vi "EcoSense.vi"() -> ()   [LabVIEW 2022 SP3]
uses:
  <vilib>/DAQmx/read.llb/DAQmx Read (Analog 1D DBL NChan 1Samp).vi
  <vilib>/DAQmx/write.llb/DAQmx Write (Digital Bool 1Line 1Point).vi
  <vilib>/DAQmx/create/channels.llb/DAQmx Create Channel (AI-Voltage-Basic).vi
  <vilib>/DAQmx/create/channels.llb/DAQmx Create Channel (DO-Digital Output).vi
  <vilib>/DAQmx/miscellaneous.llb/DAQmx Fill In Error Info.vi
panel:
  in  "Connect":bool
  in  "Write":bool
  in  "Read":bool
  in  "Exit":bool
  out "Return":string
  in  "byte count":u32
  in  "Command":string
  in  "VISA resource name":refnum<visa-resource-name>
  in  "lines 4 fire detection call":tag
  out "elapsed time":dbl
  out "PPM Meter":dbl(knob) scale=0.0..3000.0
  out "LP gas":bool
  out "CO2 gas":bool
  out "Low Temperature":bool
  out "Normal Temperature":bool
  out "HIgh Temperature":bool
  out "time":string
  out "date":string
  out "Exhaust Fan":bool
  out "Thermometer":dbl(slide) scale=0.0..100.0
  out "Temperature7 (C)":dbl
  in  "lines 3 Gas leakage call":tag
  in  "Manual Exhaust fan Switch":bool
  in  "Manual window close\n switch":bool
  out "rain":bool
  in  "lines 2 Rain sensor":tag
  out "Sensor in the bedroom 2":string
  out "Sensor in the master bedroom":string
  out "Sensor in the dining room":string
  out "Sensor in the living room":string
  out "Sensor in the kitchen":string
  in  "Manual Pump motor switch":bool
  out "Gas sensor6-(ppm)":dbl
  out "Fire":bool
  out "Gas Indicator":string
  out "Rain Sensor":dbl
  in  "lines 1 for Exhaust Fan":tag
  in  "lines 0 for Fire sensor":tag
  out "IRsensor5-Blue":dbl
  out "IR sensor1-Purple":dbl
  out "Irsensor4-Yellow":dbl
  out "IRsensor2-Green":dbl
  out "IRsensor0 - Orange":dbl
  in  "stop":bool
  in  "physical channels":tag
  # "Automated Home Wellness System"
  # "Fire Sensor"
  # "Gas Sensor"
  # "DC Power Supply"
  # "Gas Sensor6 - ppm"
  # "Thermometer"
  # "Exhuast Fan"
  # "Rain sensor indicator 3"
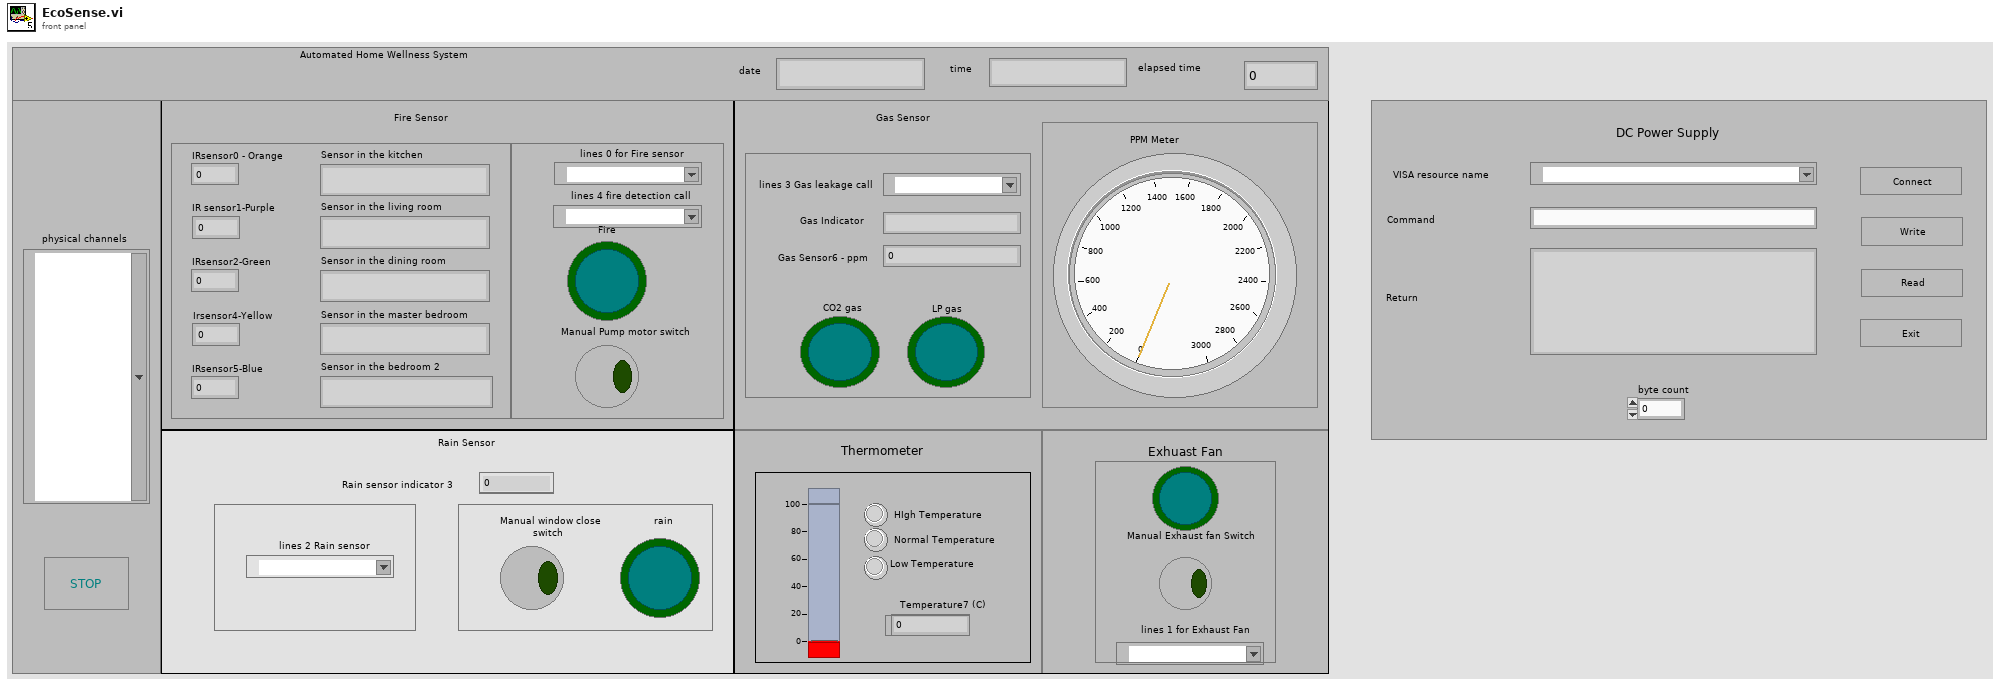
[diagram p1: front panel]
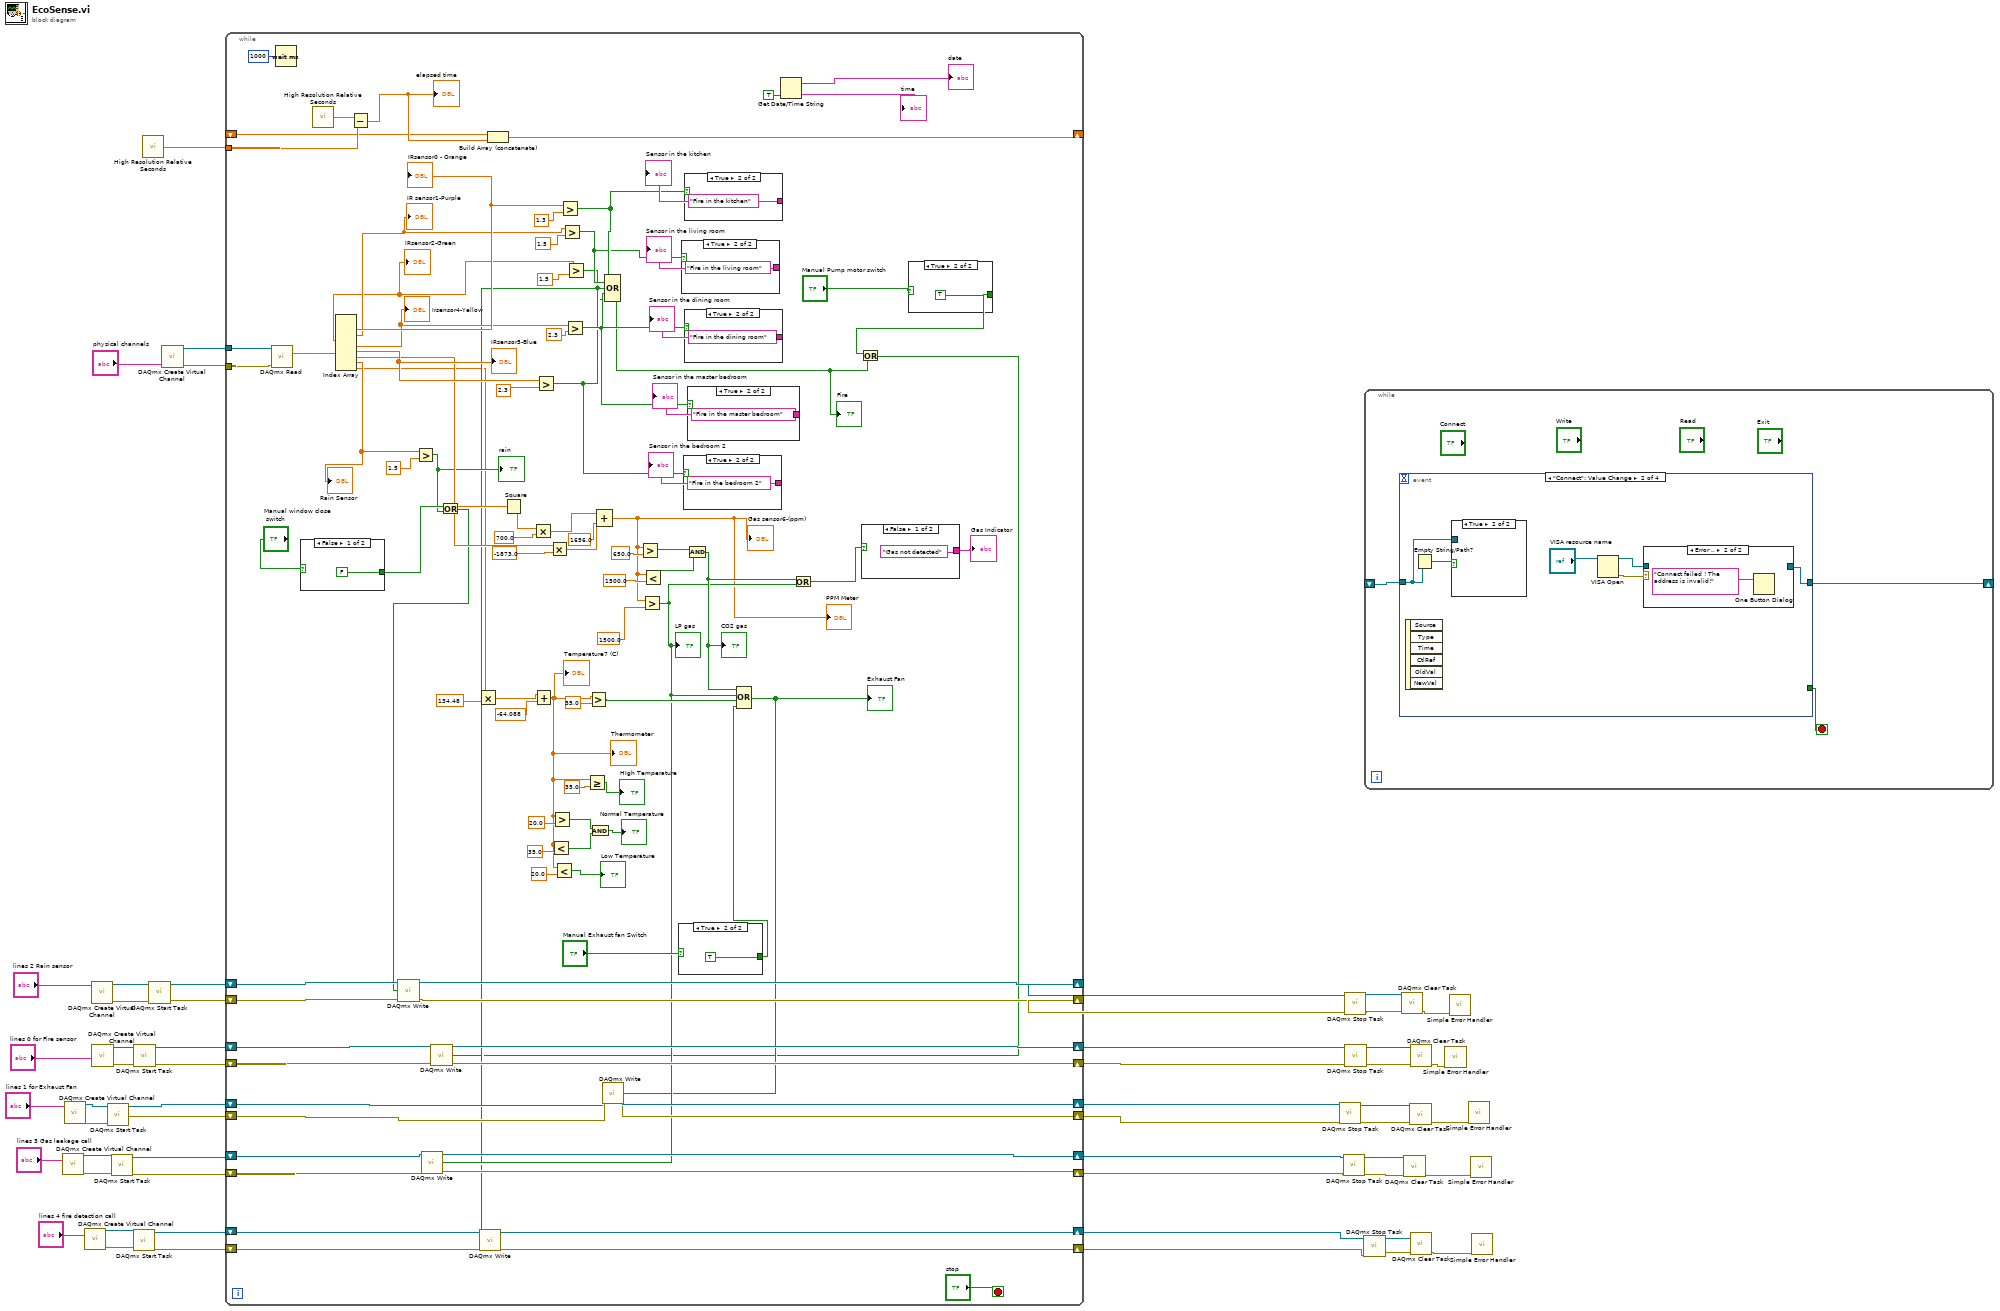
[diagram p0: block diagram]
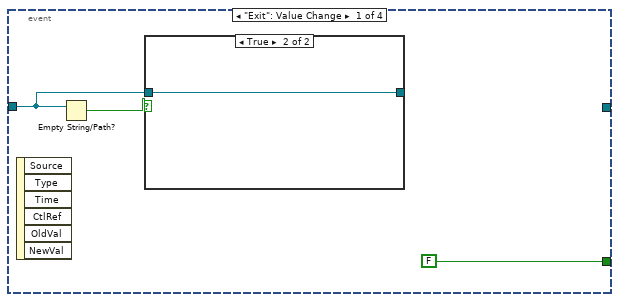
[diagram p2: hidden frame]
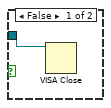
[diagram p5: hidden frame]
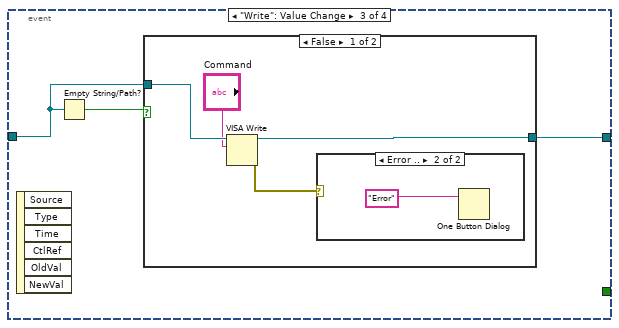
[diagram p6: hidden frame]
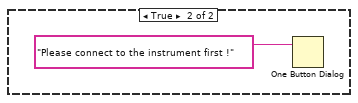
[diagram p8: hidden frame]
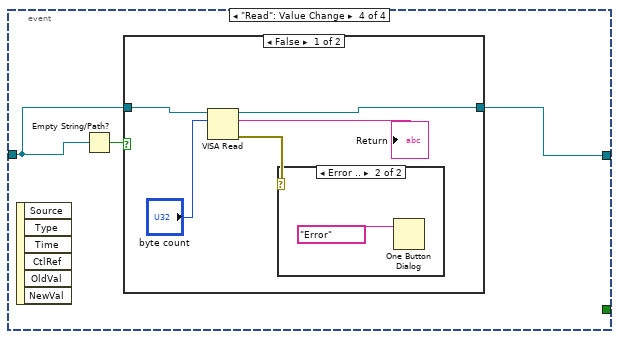
[diagram p9: hidden frame]
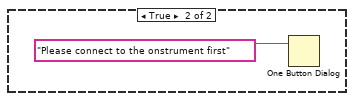
[diagram p11: hidden frame]
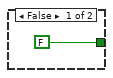
[diagram p12: hidden frame]
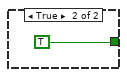
[diagram p13: hidden frame]
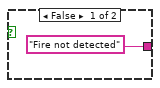
[diagram p14: hidden frame]
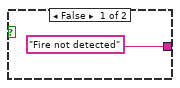
[diagram p15: hidden frame]
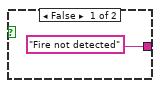
[diagram p16: hidden frame]
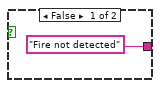
[diagram p17: hidden frame]
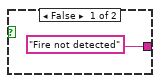
[diagram p18: hidden frame]
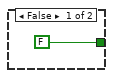
[diagram p19: hidden frame]
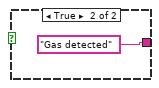
[diagram p20: hidden frame]
diagram:
  n1 = call-poly <vilib>:"DAQmx Create Virtual Channel.vi"("lines"="lines 3 Gas leakage call") -> ("task out"=w19:refnum<k21>, "error out"=w18:errorcluster)  [unwired: 13 in]
  n2 = call-poly <vilib>:"DAQmx Create Virtual Channel.vi"("lines"="lines 1 for Exhaust Fan") -> ("task out"=w43:refnum<k21>, "error out"=w27:errorcluster)  [unwired: 13 in]
  n3 = call-poly <vilib>:"DAQmx Create Virtual Channel.vi"("lines"="lines 4 fire detection call") -> ("task out"=w9:refnum<k21>, "error out"=w8:errorcluster)  [unwired: 13 in]
  n4 = call-poly <vilib>:"DAQmx Create Virtual Channel.vi"("lines"="lines 2 Rain sensor") -> ("task out"=w32:refnum<k21>, "error out"=w29:errorcluster)  [unwired: 13 in]
  n5 = call-poly <vilib>:"DAQmx Create Virtual Channel.vi"("lines"="lines 0 for Fire sensor") -> ("task out"=w50:refnum<k21>, "error out"=w28:errorcluster)  [unwired: 13 in]
  n6 = call <vilib>:"DAQmx Start Task.vi"("task/channels in"=w43, "error in"=w27) -> ("task out"=w41:refnum<k21>, "error out"=w42:errorcluster)  [unwired: 12 in]
  n7 = call <vilib>:"DAQmx Start Task.vi"("task/channels in"=w19, "error in"=w18) -> ("task out"=w17:refnum<k21>, "error out"=w16:errorcluster)  [unwired: 12 in]
  n8 = call <vilib>:"DAQmx Start Task.vi"("task/channels in"=w9, "error in"=w8) -> ("task out"=w7:refnum<k21>, "error out"=w6:errorcluster)  [unwired: 12 in]
  n9 = call <vilib>:"DAQmx Start Task.vi"("task/channels in"=w50, "error in"=w28) -> ("task out"=w46:refnum<k21>, "error out"=w35:errorcluster)  [unwired: 12 in]
  n10 = call <vilib>:"High Resolution Relative Seconds.vi"() -> ("relative seconds"=w34:dbl)
  n11 = call <vilib>:"DAQmx Start Task.vi"("task/channels in"=w32, "error in"=w29) -> ("task out"=w31:refnum<k21>, "error out"=w30:errorcluster)  [unwired: 12 in]
  n12 = call-poly <vilib>:"DAQmx Create Virtual Channel.vi"("physical channels"="physical channels") -> ("task out"=w52:refnum<k21>, "error out"=w53:errorcluster)  [unwired: 13 in]
  n13 = while {
    tunnel: w53 -> [w147]
    tunnel: w52 -> [w153]
    tunnel: w34 -> [w151]
    shift-right: [w146] -> _
    shift-left: _ -> [w148]
    shift-right: [w141] -> w47
    shift-left: w46 -> [w142]
    shift-right: [w139] -> w45
    shift-left: w35 -> [w140]
    shift-right: [w131] -> w40
    shift-left: w41 -> [w128]
    shift-right: [w129] -> w39
    shift-left: w42 -> [w130]
    shift-right: [w99] -> w25
    shift-left: w31 -> [w100]
    shift-right: [w97] -> w26
    shift-left: w30 -> [w98]
    shift-right: [w81] -> w15
    shift-left: w17 -> [w82]
    shift-right: [w80] -> w14
    shift-left: w16 -> [w83]
    shift-right: [w61] -> w5
    shift-left: w7 -> [w63]
    shift-right: [w60] -> w1
    shift-left: w6 -> [w62]
    stop <- "stop" stop-if-true
    n14 = call-poly <vilib>:"DAQmx Read.vi"("task/channels in"=w153, "error in"=w147) -> ("data"=w145:dbl[])  [unwired: 11 in, 2 out]
    n15 = Wait (ms)(milliseconds to wait=u32 1000) -> ()  [unwired: 1 out]
    n16 = case shown="False" "Manual window close\n switch" {
      tunnel: [FALSE TRUE] -> w95
      frame False {
      }
      frame True {
      }
    }
    n17 = call <vilib>:"High Resolution Relative Seconds.vi"() -> ("relative seconds"=w150:dbl)
    n18 = Index Array(array=w145) -> (element #1=w144:dbl, element #2=w137:dbl, element #3=w57:dbl, element #4=w134:dbl, element #5=w132:dbl, element #6=w117:dbl, element #7=w96:dbl, element #8=w56:dbl)  [unwired: 8 in]
    "IRsensor0 - Orange" <- w144
    "IR sensor1-Purple" <- w137
    "IRsensor5-Blue" <- w132
    "IRsensor2-Green" <- w57
    "Irsensor4-Yellow" <- w134
    "Rain Sensor" <- w96
    n19 = Subtract(x=w150, y=w151) -> (x-y=w149:dbl)
    "elapsed time" <- w149
    n20 = Greater?(x=w96, y=1.5) -> (0:w66:bool)
    "rain" <- w66
    n21 = Or(x=w95, y=w66) -> (x .or. y?=w93:bool)
    n22 = call-poly <vilib>:"DAQmx Write.vi"("task/channels in"=w100, "data"=w93, "error in"=w98) -> ("task out"=w99:refnum<k21>, "error out"=w97:errorcluster)  [unwired: 10 in, 1 out]
    n23 = Multiply(x=w56, y=134.48) -> (x*y=w91:dbl)
    n24 = Build Array (concatenate)(w148, w149) -> (w146:dbl[])
    n25 = Square(x=w117) -> (x^2=w122:dbl)
    n26 = Multiply(x=w122, y=700.0) -> (x*y=w115:dbl)
    n27 = Add(x=w91, y=-64.088) -> (x+y=w55:dbl)
    "Temperature7 (C)" <- w55
    "Thermometer" <- w55
    n28 = Greater?(x=w132, y=2.3) -> (0:w101:bool)
    n29 = Multiply(x=w117, y=-1873.0) -> (x*y=w114:dbl)
    n30 = Less?(x=w55, y=35.0) -> (x < y?=w70:bool)
    n31 = Greater?(x=w55, y=20.0) -> (0:w71:bool)
    n32 = Less?(x=w55, y=20.0) -> (x < y?=→"Low Temperature":bool)
    n33 = Greater?(x=w144, y=1.3) -> (0:w108:bool)
    n34 = Greater?(x=w137, y=1.5) -> (0:w107:bool)
    n35 = Greater?(x=w134, y=2.3) -> (0:w103:bool)
    n36 = Greater?(x=w57, y=1.5) -> (0:w105:bool)
    n37 = Greater Or Equal?(x=w55, y=35.0) -> (x >= y?=→"HIgh Temperature":bool)
    n38 = Greater?(x=w55, y=35.0) -> (0:w88:bool)
    n39 = And(x=w71, y=w70) -> (x .and. y?=→"Normal Temperature":bool)
    n40 = Compound Arithmetic op=ADD(w115, w114, 1656.0 ("value")) -> (w65:dbl)
    "Gas sensor6-(ppm)" <- w65
    "PPM Meter" <- w65
    n41 = Compound Arithmetic op=OR(w108, w107, w105, w103, w101) -> (w59:bool)
    "Fire" <- w59
    n42 = call-poly <vilib>:"DAQmx Write.vi"("task/channels in"=w63, "data"=w59, "error in"=w62) -> ("task out"=w61:refnum<k21>, "error out"=w60:errorcluster)  [unwired: 10 in, 1 out]
    n43 = Greater?(x=w65, y=650.0) -> (0:w127:bool)
    n44 = Greater?(x=w65, y=1500.0) -> (0:w79:bool)
    "LP gas" <- w79
    n45 = call-poly <vilib>:"DAQmx Write.vi"("task/channels in"=w82, "data"=w79, "error in"=w83) -> ("task out"=w81:refnum<k21>, "error out"=w80:errorcluster)  [unwired: 10 in, 1 out]
    n46 = Less?(x=w65, y=1500.0) -> (x < y?=w126:bool)
    n47 = case shown="True" "Manual Exhaust fan Switch" {
      tunnel: [FALSE TRUE] -> w86
      frame False {
      }
      frame True {
      }
    }
    n48 = case shown="True" w107 {
      tunnel: ["Fire not detected" "Fire in the living room"] -> w109
      frame False {
      }
      frame True {
      }
    }
    "Sensor in the living room" <- w109
    n49 = case shown="True" w101 {
      tunnel: ["Fire not detected" "Fire in the bedroom 2"] -> w102
      frame False {
      }
      frame True {
      }
    }
    "Sensor in the bedroom 2" <- w102
    n50 = case shown="True" w105 {
      tunnel: ["Fire not detected" "Fire in the dining room"] -> w106
      frame False {
      }
      frame True {
      }
    }
    "Sensor in the dining room" <- w106
    n51 = case shown="True" w108 {
      tunnel: ["Fire not detected" "Fire in the kitchen"] -> w110
      frame False {
      }
      frame True {
      }
    }
    "Sensor in the kitchen" <- w110
    n52 = And(x=w127, y=w126) -> (x .and. y?=w85:bool)
    "CO2 gas" <- w85
    n53 = case shown="True" w103 {
      tunnel: ["Fire not detected" "Fire in the master bedroom"] -> w104
      frame False {
      }
      frame True {
      }
    }
    "Sensor in the master bedroom" <- w104
    n54 = Compound Arithmetic op=OR(w85, w79, w88, w86) -> (w64:bool)
    "Exhaust Fan" <- w64
    n55 = call-poly <vilib>:"DAQmx Write.vi"("task/channels in"=w128, "data"=w64, "error in"=w130) -> ("task out"=w131:refnum<k21>, "error out"=w129:errorcluster)  [unwired: 10 in, 1 out]
    n56 = Get Date/Time String(want seconds? (F)=TRUE) -> (date string=→"date":string, time string=→"time":string)  [unwired: 2 in]
    n57 = Or(x=w85, y=w79) -> (x .or. y?=w84:bool)
    n58 = case shown="False" w84 {
      tunnel: ["Gas not detected" "Gas detected"] -> w124
      frame False {
      }
      frame True {
      }
    }
    "Gas Indicator" <- w124
    n59 = case shown="True" "Manual Pump motor switch" {
      tunnel: [FALSE TRUE] -> w111
      frame False {
      }
      frame True {
      }
    }
    n60 = Or(x=w111, y=w59) -> (x .or. y?=w58:bool)
    n61 = call-poly <vilib>:"DAQmx Write.vi"("task/channels in"=w142, "data"=w58, "error in"=w140) -> ("task out"=w141:refnum<k21>, "error out"=w139:errorcluster)  [unwired: 10 in, 1 out]
  }
  n62 = call <vilib>:"DAQmx Stop Task.vi"("task/channels in"=w40, "error in"=w39) -> ("task out"=w38:refnum<k21>, "error out"=w37:errorcluster)  [unwired: 12 in]
  n63 = call <vilib>:"DAQmx Stop Task.vi"("task/channels in"=w15, "error in"=w14) -> ("task out"=w13:refnum<k21>, "error out"=w12:errorcluster)  [unwired: 12 in]
  n64 = call <vilib>:"DAQmx Stop Task.vi"("task/channels in"=w25, "error in"=w26) -> ("task out"=w22:refnum<k21>, "error out"=w24:errorcluster)  [unwired: 12 in]
  n65 = call <vilib>:"DAQmx Stop Task.vi"("task/channels in"=w47, "error in"=w45) -> ("task out"=w49:refnum<k21>, "error out"=w48:errorcluster)  [unwired: 12 in]
  n66 = call <vilib>:"DAQmx Stop Task.vi"("task/channels in"=w5, "error in"=w1) -> ("task out"=w4:refnum<k21>, "error out"=w2:errorcluster)  [unwired: 12 in]
  n67 = while {
    shift-right: [w173] -> _
    shift-left: _ -> [w174]
    stop <- w172 stop-if-true
    n68 = event shown="[1] \"Connect\": Value Change" {
      selector: _ -> [_ _ _ _]
      dyn-events: _ -> [_ _ _ _]
      timeout: _ -> [_ _ _ _]
      tunnel: w174 -> [w176 w182 w190 w199]
      tunnel: [_ w180 w189 w198] -> w173
      tunnel: [FALSE _ _ _] -> w172
      event "Exit": Value Change {
        n69 = event-data() -> ()  [unwired: 1 in, 6 out]
        n70 = Empty String/Path?(string/path=w176) -> (empty?=w177:bool)
        n71 = case shown="True" w177 {
          tunnel: w176 -> [w178 w179]
          tunnel: [w178 w179] -> _
          frame False {
          }
          frame True {
          }
        }
      }
      event "Connect": Value Change {
        n72 = event-data() -> ()  [unwired: 1 in, 6 out]
        n73 = Empty String/Path?(string/path=w182) -> (empty?=w183:bool)
        n74 = case shown="True" w183 {
          tunnel: w182 -> [w188 _]
          frame False {
            n75 = VISA Close(VISA resource name=w188) -> ()  [unwired: 1 in, 1 out]
          }
          frame True {
          }
        }
        n76 = VISA Open(VISA resource name="VISA resource name") -> (VISA resource name=w181:refnum<visa-resource-name>, error out=w184:errorcluster)  [unwired: 4 in]
        n77 = case shown="Error .." w184 {
          tunnel: w181 -> [w186 _]
          tunnel: [w186 _] -> w180
          frame No Error {
          }
          frame Error {
            n78 = One Button Dialog(message="Connect failed ! The address is invalid!") -> ()  [unwired: 1 in, 1 out]
          }
        }
      }
      event "Write": Value Change {
        n79 = event-data() -> ()  [unwired: 1 in, 6 out]
        n80 = Empty String/Path?(string/path=w190) -> (empty?=w191:bool)
        n81 = case shown="False" w191 {
          tunnel: w190 -> [w195 _]
          tunnel: [w194 _] -> w189
          frame False {
            n82 = VISA Write(VISA resource name=w195, write buffer="Command") -> (VISA resource name out=w194:refnum<visa-resource-name>, error out=w192:errorcluster)  [unwired: 1 in, 1 out]
            n83 = case shown="Error .." w192 {
              frame No Error {
              }
              frame Error {
                n84 = One Button Dialog(message="Error") -> ()  [unwired: 1 in, 1 out]
              }
            }
          }
          frame True {
            n85 = One Button Dialog(message="Please connect to the instrument first !") -> ()  [unwired: 1 in, 1 out]
          }
        }
      }
      event "Read": Value Change {
        n86 = event-data() -> ()  [unwired: 1 in, 6 out]
        n87 = Empty String/Path?(string/path=w199) -> (empty?=w200:bool)
        n88 = case shown="False" w200 {
          tunnel: w199 -> [w205 _]
          tunnel: [w204 _] -> w198
          frame False {
            n89 = VISA Read(VISA resource name=w205, byte count="byte count") -> (VISA resource name out=w204:refnum<visa-resource-name>, read buffer=→"Return":string, error out=w202:errorcluster)  [unwired: 1 in, 1 out]
            n90 = case shown="Error .." w202 {
              frame No Error {
              }
              frame Error {
                n91 = One Button Dialog(message="Error") -> ()  [unwired: 1 in, 1 out]
              }
            }
          }
          frame True {
            n92 = One Button Dialog(message="Please connect to the onstrument first") -> ()  [unwired: 1 in, 1 out]
          }
        }
      }
    }
  }
  n93 = call <vilib>:"DAQmx Clear Task.vi"("task in"=w22, "error in"=w24) -> ("error out"=w23:errorcluster)  [unwired: 13 in]
  n94 = call <vilib>:"DAQmx Clear Task.vi"("task in"=w13, "error in"=w12) -> ("error out"=w11:errorcluster)  [unwired: 13 in]
  n95 = call <vilib>:"DAQmx Clear Task.vi"("task in"=w38, "error in"=w37) -> ("error out"=w21:errorcluster)  [unwired: 13 in]
  n96 = call <vilib>:"DAQmx Clear Task.vi"("task in"=w49, "error in"=w48) -> ("error out"=w44:errorcluster)  [unwired: 13 in]
  n97 = call <vilib>:"DAQmx Clear Task.vi"("task in"=w4, "error in"=w2) -> ("error out"=w3:errorcluster)  [unwired: 13 in]
  n98 = call <vilib>:"Simple Error Handler.vi"("error in (no error)"=w44) -> ()  [unwired: 4 in, 5 out]
  n99 = call <vilib>:"Simple Error Handler.vi"("error in (no error)"=w23) -> ()  [unwired: 4 in, 5 out]
  n100 = call <vilib>:"Simple Error Handler.vi"("error in (no error)"=w21) -> ()  [unwired: 4 in, 5 out]
  n101 = call <vilib>:"Simple Error Handler.vi"("error in (no error)"=w11) -> ()  [unwired: 4 in, 5 out]
  n102 = call <vilib>:"Simple Error Handler.vi"("error in (no error)"=w3) -> ()  [unwired: 4 in, 5 out]
